vi "Update Methods Registration.vi"(8 "error in (no error)":errorcluster, 11 "Server class in":refnum<vi>) -> (0 "error out":errorcluster, 3 "Server class out":refnum<vi>)   [LabVIEW 2019, in "gRPC Scripting Tools.lvlib"]
uses:
  gRPC Scripting Tools.lvlib
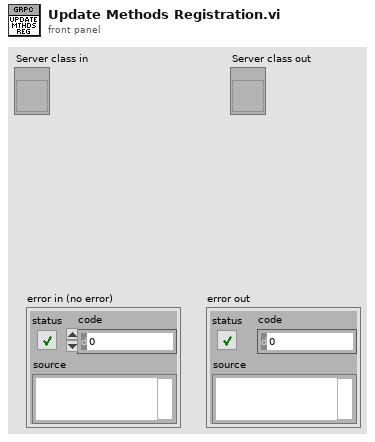
[diagram p1: front panel]
types:
  T1 = typedef "LVPointTypeDef.ctl" = cluster{"Horizontal":i16, "Vertical":i16}
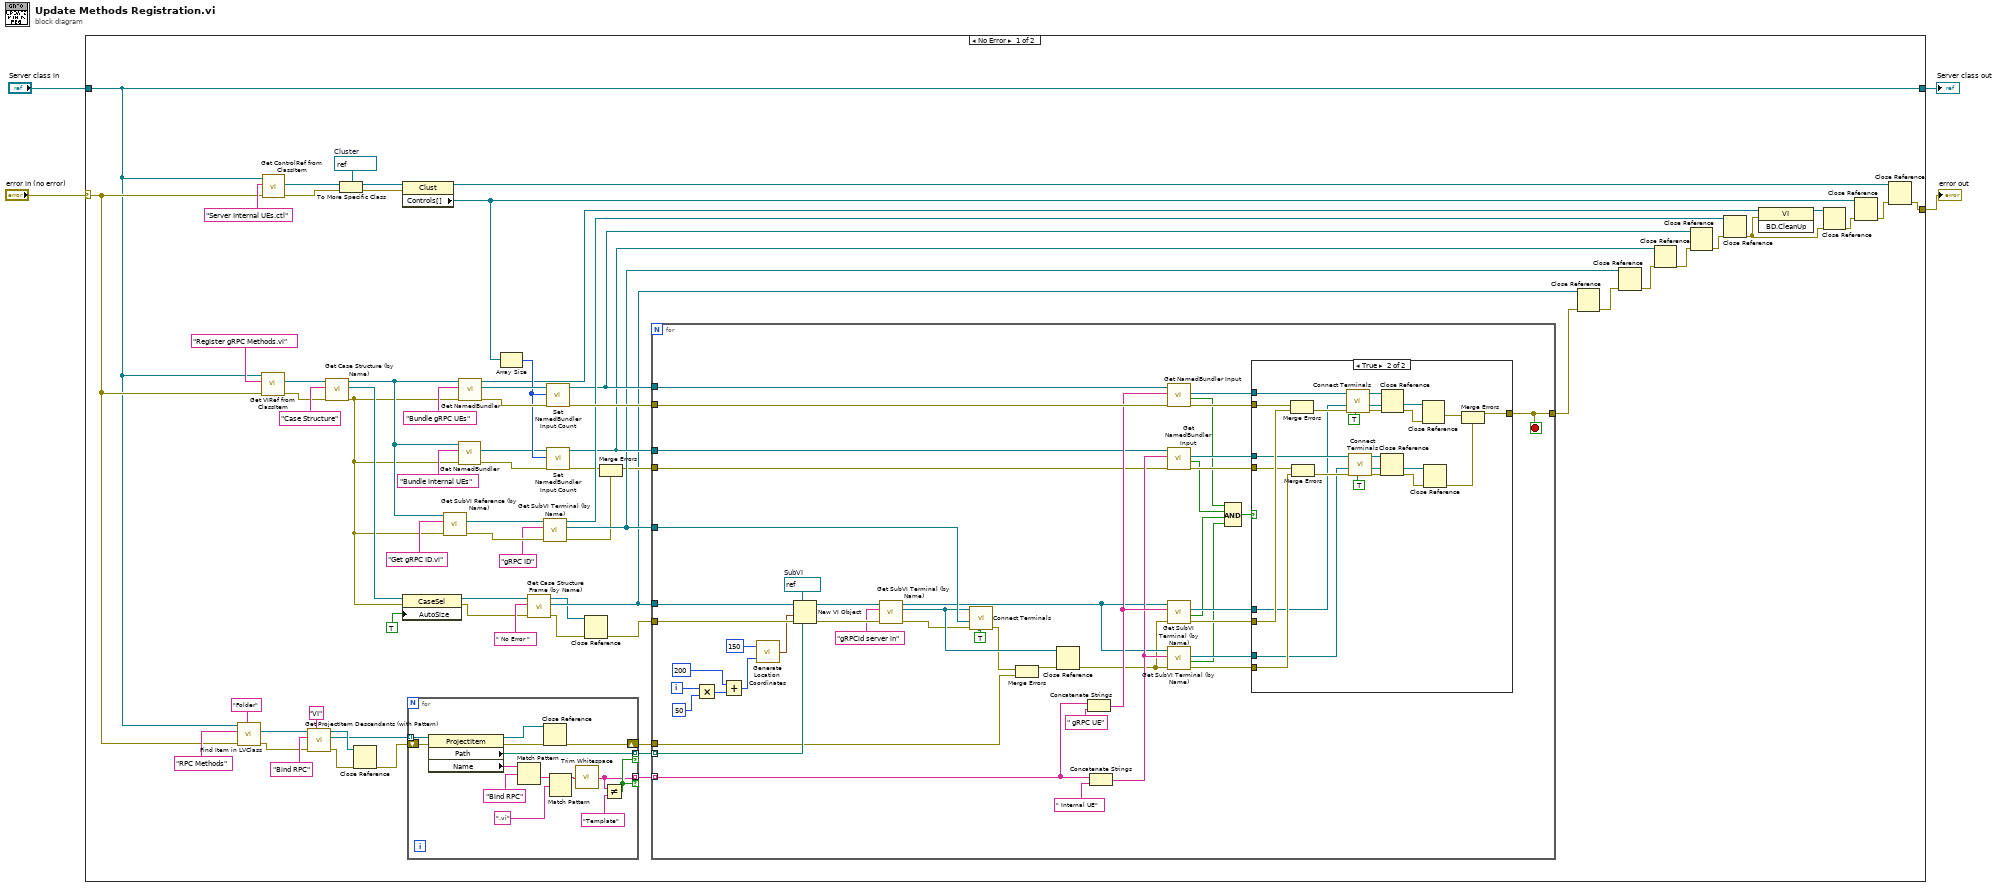
[diagram p0: block diagram]
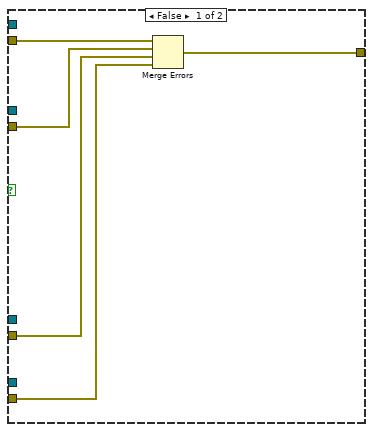
[diagram p2: hidden frame]
diagram:
  n1 = case shown="No Error" "error in (no error)" {
    selector: "error in (no error)" -> [w27 w157]
    tunnel: [w13 w157] -> w4
    tunnel: "Server class in" -> [w26 w158]
    tunnel: [w26 w158] -> w1
    frame No Error {
      w64 = refnum<vi> refnum  # Cluster
      n2 = call "Find Item in LVClass.vi"("Item Type"="Folder", "error in (no error)"=w27, "Item Name"="RPC Methods", "Class Item in"=w26) -> ("error out"=w38:errorcluster, "Project Item (Class Item)"=w39:refnum<vi>)  [unwired: 4 in, 2 out]
      n3 = call "Get VIRef from ClassItem.vi"("error in (no error)"=w27, "Item Name"="Register gRPC Methods.vi", "LVClassLibrary in"=w26) -> ("error out"=w58:errorcluster, "VIref out"=w71:refnum<vi>)  [unwired: 5 in, 2 out]
      n4 = call "Get ControlRef from ClassItem.vi"("error in (no error)"=w27, "Item Name"="Server Internal UEs.ctl", "LVClassLibrary in"=w26) -> ("error out"=w65:errorcluster, "Control ref out"=w63:refnum<vi>)  [unwired: 5 in, 2 out]
      n5 = call "Get ProjectItem Descendants (with Pattern).vi"("Type"="VI", "error in (no error)"=w38, "Pattern"="Bind RPC" ("regular expression"), "ProjectItem in"=w39) -> ("error out"=w37:errorcluster, "ProjectItem descendents"=w12:refnum<vi>[], "ProjectItem out"=w35:refnum<vi>)  [unwired: 5 in]
      n6 = call "Get Case Structure (by Name).vi"("error in (no error)"=w58, "Case Structure name"="Case Structure" ("y"), "VI ref in"=w71) -> ("error out"=w16:errorcluster, "CaseStructure out"=w20:refnum<vi>, "VI ref out"=w48:refnum<vi>)  [unwired: 5 in, 1 out]
      n7 = To More Specific Class(target class=w64, reference=w63, error in=w65) -> (specific class reference=w66:refnum<vi>, error out=w68:errorcluster)
      n8 = Close Reference(reference=w35, error in (no error)=w37) -> (error out=w9:errorcluster)
      n9 = property class="Clust"(reference=w66, error in=w68) -> (reference out=w15:refnum<vi>, "Controls[]"=w67:refnum<vi>[])  [unwired: 1 out]
      n10 = property class="CaseSel"(reference=w20, error in=w16, "AutoSize"=TRUE ("AutoSize To Fit Contents?")) -> (reference out=w19:refnum<vi>, error out=w18:errorcluster)
      n11 = for {
        tunnel: w12 -> [w86] mode=indexing
        tunnel: [w73] -> w10 mode=indexing if=w79
        tunnel: [w80] -> w11 mode=indexing if=w79
        shift-right: [w75] -> w8
        shift-left: w9 -> [w76]
        n12 = property class="ProjectItem"(reference=w86, error in=w76) -> (reference out=w77:refnum<vi>, error out=w78:errorcluster, "Path"=w80:path, "Name"=w82:string)
        n13 = Match Pattern(string=w82, regular expression="Bind RPC") -> (after substring=w84:string)  [unwired: 1 in, 3 out]
        n14 = Close Reference(reference=w77, error in (no error)=w78) -> (error out=w75:errorcluster)
        n15 = Match Pattern(string=w84, regular expression=".vi") -> (before substring=w74:string)  [unwired: 1 in, 3 out]
        n16 = call <vilib>:"Trim Whitespace.vi"("string"=w74) -> ("trimmed string"=w73:string)  [unwired: 1 in]
        n17 = Not Equal?(x=w73, y="Template") -> (x != y?=w79:bool)
      }
      n18 = call "Get SubVI Reference (by Name).vi"("error in (no error)"=w16, "SubVI Name"="Get gRPC ID.vi", "Owner VI in"=w48) -> ("error out"=w45:errorcluster, "SubVI Refnum out"=w46:refnum<vi>)  [unwired: 5 in, 2 out]
      n19 = call "Get NamedBundler.vi"("error in (no error)"=w16, "Label"="Bundle Internal UEs" ("name/order"), "Owner VI in"=w48) -> ("error out"=w49:errorcluster, "NamedBundler ref out"=w50:refnum<vi>)  [unwired: 5 in, 2 out]
      n20 = call "Get NamedBundler.vi"("error in (no error)"=w16, "Label"="Bundle gRPC UEs" ("name/order"), "Owner VI in"=w48) -> ("error out"=w52:errorcluster, "NamedBundler ref out"=w70:refnum<vi>, "Owner VI out"=w7:refnum<vi>)  [unwired: 5 in, 1 out]
      n21 = Array Size(array=w67) -> (size(s)=w51:i32)
      n22 = call "Get Case Structure Frame (by Name).vi"("error in (no error)"=w18, "element"=" No Error ", "CaseStructure in"=w19) -> ("error out"=w36:errorcluster, "Frame ref out"=w22:refnum<vi>, "CaseStructure out"=w21:refnum<vi>)  [unwired: 5 in, 1 out]
      n23 = call "Get SubVI Terminal (by Name).vi"("error in (no error)"=w45, "Terminal name"="gRPC ID", "SubVI in"=w46) -> ("error out"=w24:errorcluster, "SubVI Term ref"=w34:refnum<vi>, "SubVI out"=w43:refnum<vi>)  [unwired: 5 in, 1 out]
      n24 = call "Set NamedBundler Input Count.vi"("error in (no error)"=w52, "Numeric"=w51, "NamedBundler in"=w70) -> ("error out"=w60:errorcluster, "NamedBundler out"=w41:refnum<vi>)  [unwired: 7 in]
      n25 = call "Set NamedBundler Input Count.vi"("error in (no error)"=w49, "Numeric"=w51, "NamedBundler in"=w50) -> ("error out"=w25:errorcluster, "NamedBundler out"=w40:refnum<vi>)  [unwired: 7 in]
      n26 = Close Reference(reference=w21, error in (no error)=w36) -> (error out=w42:errorcluster)
      n27 = Merge Errors(w25, w24) -> (w23:errorcluster)
      n28 = for {
        tunnel: w22 -> [w132]
        tunnel: w60 -> [w131]
        tunnel: w41 -> [w130]
        tunnel: w42 -> [w124]
        tunnel: w23 -> [w120]
        tunnel: w40 -> [w121]
        tunnel: [w113] -> w33
        tunnel: w34 -> [w104]
        tunnel: w11 -> [w89] mode=indexing
        tunnel: w10 -> [w87] mode=indexing
        tunnel: w8 -> [w88]
        i -> [w101]
        stop <- w113 stop-if-true
        w129 = refnum<vi> refnum  # SubVI
        n29 = Multiply(x=w101, y=50) -> (x*y=w99:i32)
        n30 = Add(x=i16 200 ("Horizontal"), y=w99) -> (x+y=w97:i32)
        n31 = call "Generate Location Coordinates.vi"("Vertical"=w97, "Horizontal"=i16 150) -> ("Location out"=w96:T1)
        n32 = New VI Object(vi object class=w129, owner refnum=w132, position/next to=w96, 6:w89, 8:w124) -> (object refnum=w106:refnum<vi>, 0:w107:errorcluster)  [unwired: 3 in]
        n33 = call "Get SubVI Terminal (by Name).vi"("error in (no error)"=w107, "Terminal name"="gRPCid server in", "SubVI in"=w106) -> ("error out"=w93:errorcluster, "SubVI Term ref"=w94:refnum<vi>, "SubVI out"=w103:refnum<vi>)  [unwired: 5 in, 1 out]
        n34 = call "Connect Terminals.vi"("Auto Route? (F)"=TRUE, "Error In"=w93, "Source Terminal"=w104, "Sink Terminal"=w94) -> ("Error Out"=w91:errorcluster)  [unwired: 7 in]
        n35 = Merge Errors(w91, w88) -> (w90:errorcluster)
        n36 = Close Reference(reference=w94, error in (no error)=w90) -> (error out=w92:errorcluster)
        n37 = Concatenate Strings(w87, " gRPC UE" ("string")) -> (w125:string)
        n38 = Concatenate Strings(w87, " Internal UE" ("string")) -> (w122:string)
        n39 = call "Get NamedBundler Input.vi"("error in (no error)"=w131, "Input name"=w125, "NamedBundler ref in"=w130) -> ("error out"=w117:errorcluster, "Found?"=w112:bool, "Input Term ref"=w128:refnum<vi>)  [unwired: 5 in, 1 out]
        n40 = call "Get NamedBundler Input.vi"("error in (no error)"=w120, "Input name"=w122, "NamedBundler ref in"=w121) -> ("error out"=w115:errorcluster, "Found?"=w111:bool, "Input Term ref"=w119:refnum<vi>)  [unwired: 5 in, 1 out]
        n41 = call "Get SubVI Terminal (by Name).vi"("error in (no error)"=w92, "Terminal name"=w125, "SubVI in"=w103) -> ("error out"=w116:errorcluster, "Found?"=w110:bool, "SubVI Term ref"=w127:refnum<vi>)  [unwired: 5 in, 1 out]
        n42 = call "Get SubVI Terminal (by Name).vi"("error in (no error)"=w92, "Terminal name"=w122, "SubVI in"=w103) -> ("error out"=w114:errorcluster, "Found?"=w109:bool, "SubVI Term ref"=w118:refnum<vi>)  [unwired: 5 in, 1 out]
        n43 = Compound Arithmetic op=AND(w112, w111, w110, w109) -> (w108:bool)
        n44 = case shown="True" w108 {
          tunnel: w128 -> [_ w144]
          tunnel: w127 -> [_ w142]
          tunnel: w119 -> [_ w146]
          tunnel: w118 -> [_ w141]
          tunnel: w117 -> [w137 w156]
          tunnel: w116 -> [w134 w155]
          tunnel: w115 -> [w135 w154]
          tunnel: w114 -> [w133 w153]
          tunnel: [w136 w150] -> w113
          frame False {
            n45 = Merge Errors(w137, w135, w134, w133) -> (w136:errorcluster)
          }
          frame True {
            n46 = Merge Errors(w156, w155) -> (w152:errorcluster)
            n47 = Merge Errors(w154, w153) -> (w151:errorcluster)
            n48 = call "Connect Terminals.vi"("Auto Route? (F)"=TRUE, "Error In"=w152, "Source Terminal"=w142, "Sink Terminal"=w144) -> ("Error Out"=w145:errorcluster)  [unwired: 7 in]
            n49 = call "Connect Terminals.vi"("Auto Route? (F)"=TRUE, "Error In"=w151, "Source Terminal"=w141, "Sink Terminal"=w146) -> ("Error Out"=w147:errorcluster)  [unwired: 7 in]
            n50 = Close Reference(reference=w146, error in (no error)=w147) -> (error out=w140:errorcluster)
            n51 = Close Reference(reference=w144, error in (no error)=w145) -> (error out=w143:errorcluster)
            n52 = Close Reference(reference=w142, error in (no error)=w143) -> (error out=w139:errorcluster)
            n53 = Close Reference(reference=w141, error in (no error)=w140) -> (error out=w138:errorcluster)
            n54 = Merge Errors(w139, w138) -> (w150:errorcluster)
          }
        }
      }
      n55 = Close Reference(reference=w22, error in (no error)=w33) -> (error out=w32:errorcluster)
      n56 = Close Reference(reference=w34, error in (no error)=w32) -> (error out=w31:errorcluster)
      n57 = Close Reference(reference=w40, error in (no error)=w31) -> (error out=w30:errorcluster)
      n58 = Close Reference(reference=w41, error in (no error)=w30) -> (error out=w29:errorcluster)
      n59 = Close Reference(reference=w43, error in (no error)=w29) -> (error out=w5:errorcluster)
      n60 = invoke class="VI" method="BD.CleanUp"(reference=w7, error in=w5) -> (reference out=w6:refnum<vi>)  [unwired: 1 in, 2 out]
      n61 = Close Reference(reference=w6, error in (no error)=w5) -> (error out=w28:errorcluster)
      n62 = Close Reference(reference=w67, error in (no error)=w28) -> (error out=w14:errorcluster)
      n63 = Close Reference(reference=w15, error in (no error)=w14) -> (error out=w13:errorcluster)
    }
    frame Error {
    }
  }
  "error out" <- w4
  "Server class out" <- w1
